vi "CreateSerializableDataTypedef.vi"(4 "SaveTo Path":path, 6 "Template typedef path":path, 8 "error in (no error)":errorcluster, 10 "Application":refnum<vi>, 11 "LVClassLibrary Ref":refnum<vi>) -> (0 "error out":errorcluster, 2 "Application":refnum<vi>, 3 "LVClassLibrary Ref":refnum<vi>)   [LabVIEW 2019, in "BlueSerializationScripts.lvlib"]
uses:
  BlueSerializationScripts.lvlib
  BlueSerialVirtualFolders.ctl
  <vilib>/Utility/miscctls.llb/LVPointTypeDef.ctl
  BlueUtilityScripts/BlueUtilityScripts.lvlib
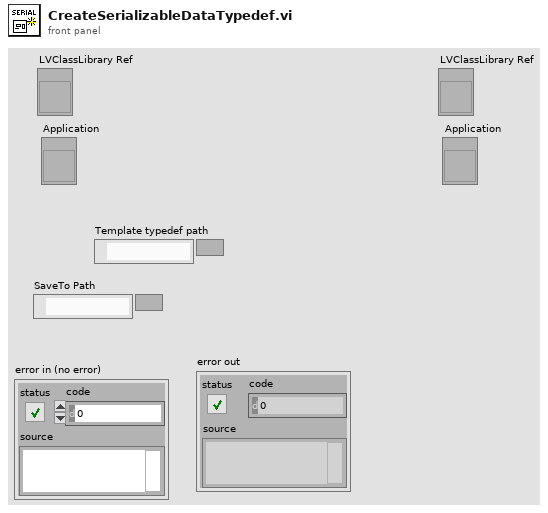
[diagram p1: front panel]
types:
  T1 = enum32{"invalid VI type", "Standard VI", "Control VI", "Global VI", "Polymorphic VI", "Configuration VI", "SubSystem", "Facade VI", "Method VI"}
  T2 = typedef "BlueSerializationScripts.lvlib/BlueSerialVirtualFolders.ctl" = enum16{"BlueSerialization", "Mutations"}
  T3 = typedef "LVPointTypeDef.ctl" = cluster{"Horizontal":i16, "Vertical":i16}
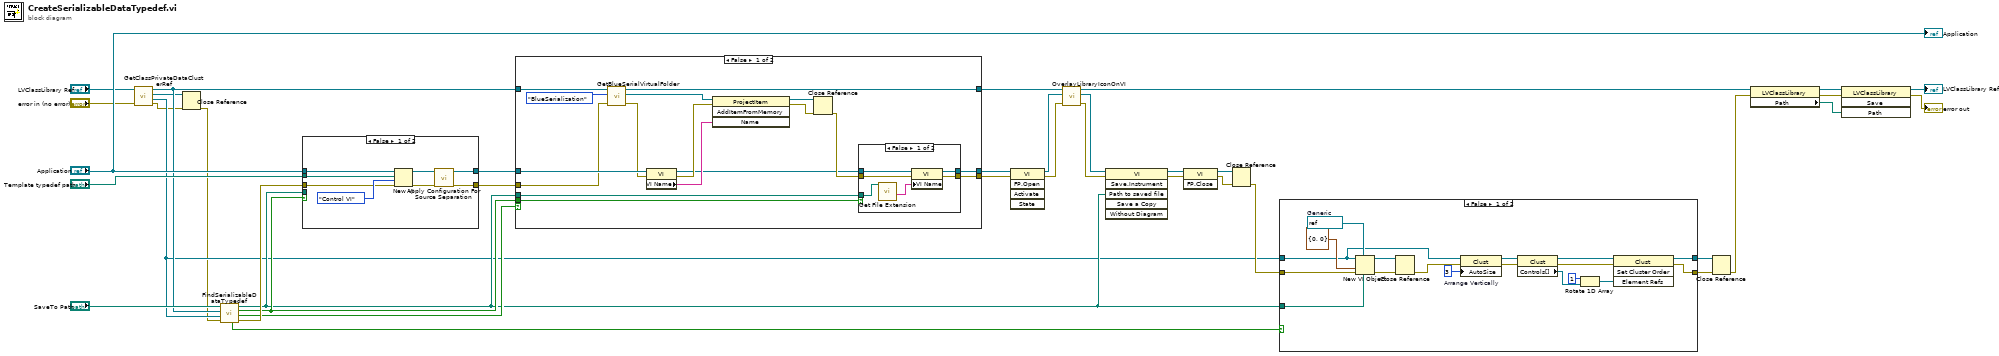
[diagram p0: block diagram]
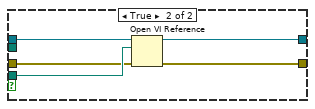
[diagram p4: hidden frame]
diagram:
  n1 = call "GetClassPrivateDataClusterRef.vi"("error in (no error)"="error in (no error)", "LVClassLibrary Ref"="LVClassLibrary Ref") -> ("error out"=w14:errorcluster, "Class private data cluster refnum"=w20:refnum<vi>, "Class private data vi refnum"=w15:refnum<vi>, "LVClassLibrary Ref"=w27:refnum<vi>)  [unwired: 6 in]
  n2 = Close Reference(reference=w15, error in (no error)=w14) -> (error out=w13:errorcluster)
  n3 = call "FindSerializableDataTypedef.vi"("error in (no error)"=w13, "Private data cluster refnum"=w20, "LVClass refnum"=w27, "SaveTo Path"="SaveTo Path") -> ("error out"=w32:errorcluster, "ctl is in class library?"=w31:bool, "ctl File exists?"=w26:bool, "SaveTo Path"=w25:path, "ctl is in private data?"=w28:bool)  [unwired: 3 in]
  n4 = case shown="False" w26 {
    tunnel: [w45 w50] -> w38
    tunnel: "Template typedef path" -> [w44 _]
    tunnel: w32 -> [w43 w47]
    tunnel: "Application" -> [w42 w51]
    tunnel: [w40 w49] -> w30
    tunnel: w25 -> [_ w48]
    frame False {
      n5 = New VI(8:w43, 9:T1."Control VI" ("vi type (standard vi)"), 10:w44, 11:w42) -> (0:w41:errorcluster, 3:w39:refnum<vi>)  [unwired: 3 out]
      n6 = call <vilib>:"Apply Configuration For Source Separation.vi"("error in (no error)"=w41, "VI in"=w39) -> ("error out"=w40:errorcluster, "VI out"=w45:refnum<vi>)  [unwired: 8 in]
    }
    frame True {
      n7 = Open VI Reference(application reference (local)=w51, vi path=w48, error in (no error)=w47) -> (vi reference=w50:refnum<vi>, error out=w49:errorcluster)  [unwired: 3 in]
    }
  }
  n8 = case shown="False" w31 {
    tunnel: [w60 w77] -> w24
    tunnel: w38 -> [w68 w77]
    tunnel: [w58 w78] -> w23
    tunnel: [w56 w79] -> w12
    tunnel: w27 -> [w57 w79]
    tunnel: w30 -> [w54 w78]
    tunnel: w26 -> [w63 _]
    tunnel: w25 -> [w59 _]
    frame False {
      n9 = call "GetBlueSerialVirtualFolder.vi"("error in (no error)"=w54, "Virtual Folder"=BlueSerialVirtualFolders."BlueSerialization", "LVClassLibrary Ref"=w57) -> ("error out"=w53:errorcluster, "Folder Refnum out"=w52:refnum<vi>, "LVClassLibrary Ref"=w56:refnum<vi>)  [unwired: 6 in]
      n10 = property class="VI"(reference=w68, error in=w53) -> (reference out=w61:refnum<vi>, error out=w65:errorcluster, "VI Name"=w64:string)
      n11 = invoke class="ProjectItem" method="AddItemFromMemory"(reference=w52, error in=w65, "Name"=w64) -> (reference out=w66:refnum<vi>, error out=w67:errorcluster)  [unwired: 1 in, 2 out]
      n12 = Close Reference(reference=w66, error in (no error)=w67) -> (error out=w62:errorcluster)
      n13 = case shown="False" w63 {
        tunnel: w62 -> [w74 w75]
        tunnel: w61 -> [w73 w76]
        tunnel: [w72 w76] -> w60
        tunnel: [w71 w75] -> w58
        tunnel: w59 -> [w69 _]
        frame False {
          n14 = call <vilib>:"Get File Extension.vi"("file"=w69) -> ("filename without extension"=w70:string)  [unwired: 6 in, 4 out]
          n15 = property class="VI"(reference=w73, error in=w74, "VI Name"=w70) -> (reference out=w72:refnum<vi>, error out=w71:errorcluster)
        }
        frame True {
        }
      }
    }
    frame True {
    }
  }
  n16 = invoke class="VI" method="FP.Open"(reference=w24, error in=w23) -> (reference out=w11:refnum<vi>, error out=w10:errorcluster)  [unwired: 3 in, 3 out]
  n17 = call "OverlayLibraryIconOnVI.vi"("error in (no error)"=w10, "VI Refnum out"=w11, "LVClassLibrary"=w12) -> ("error out"=w9:errorcluster, "VI Refnum out"=w8:refnum<vi>, "LVClassLibrary"=w6:refnum<vi>)  [unwired: 5 in, 1 out]
  n18 = invoke class="VI" method="Save.Instrument"(reference=w8, error in=w9, "Path to saved file"=w25) -> (reference out=w19:refnum<vi>, error out=w18:errorcluster)  [unwired: 3 in, 4 out]
  n19 = invoke class="VI" method="FP.Close"(reference=w19, error in=w18) -> (reference out=w17:refnum<vi>, error out=w16:errorcluster)  [unwired: 1 in, 1 out]
  n20 = Close Reference(reference=w17, error in (no error)=w16) -> (error out=w29:errorcluster)
  n21 = case shown="False" w28 {
    tunnel: [w87 w99] -> w22
    tunnel: w20 -> [w89 w98]
    tunnel: w25 -> [w97 _]
    tunnel: w29 -> [w96 w99]
    tunnel: [w88 w98] -> w21
    frame False {
      w91 = u32 3  # Arrange Vertically
      w92 = refnum<vi> refnum  # Generic
      n22 = New VI Object(vi object class=w92, owner refnum=w89, position/next to=T3 {"Horizontal"=0, "Vertical"=0} ("relative position/next to refnum"), 6:w97, 8:w96) -> (object refnum=w93:refnum<vi>, 0:w94:errorcluster)  [unwired: 3 in]
      n23 = Close Reference(reference=w93, error in (no error)=w94) -> (error out=w90:errorcluster)
      n24 = property class="Clust"(reference=w89, error in=w90, "AutoSize"=w91) -> (reference out=w86:refnum<vi>, error out=w85:errorcluster)
      n25 = property class="Clust"(reference=w86, error in=w85) -> (reference out=w84:refnum<vi>, error out=w83:errorcluster, "Controls[]"=w82:refnum<vi>[])
      n26 = Rotate 1D Array(1:w82, 2:1 ("n")) -> (0:w80:refnum<vi>[])
      n27 = invoke class="Clust" method="Set Cluster Order"(reference=w84, error in=w83, "Element Refs"=w80) -> (reference out=w88:refnum<vi>, error out=w87:errorcluster)  [unwired: 1 in, 2 out]
    }
    frame True {
    }
  }
  n28 = Close Reference(reference=w21, error in (no error)=w22) -> (error out=w2:errorcluster)
  n29 = property class="LVClassLibrary"(reference=w6, error in=w2) -> (reference out=w5:refnum<vi>, error out=w4:errorcluster, "Path"=w3:path)
  n30 = invoke class="LVClassLibrary" method="Save"(reference=w5, error in=w4, "Path"=w3) -> (reference out=→"LVClassLibrary Ref":refnum<vi>, error out=→"error out":errorcluster)  [unwired: 1 in, 2 out]
  "Application" <- "Application"
